vi "File_Application  Path INI Location.vi"() -> (0 "Path INI Location":path)   [LabVIEW 2015]
uses:
  <vilib>/Utility/sysdir.llb/System Directory Type.ctl
panel:
  in  "Name of System (Save as Default)":string="MySystem.ini"
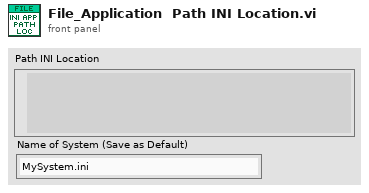
[diagram p1: front panel]
types:
  T1 = typedef "System Directory Type.ctl" = i32
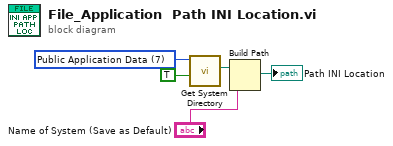
[diagram p0: block diagram]
diagram:
  w1 = T1 7 items=["User Home"=0, "User Desktop"=1, "User Documents"=2, "User Application Data"=3, "User Preferences"=4, "User Temporary"=5, "Public Documents"=6, "Public Application Data"=7, "Public Preferences"=8, "Public Cache"=13, "System Core Libraries"=9, "System Installed Libraries"=10, "Application Files"=11, "Boot Volume Root"=12] ("system directory type")
  n1 = call <vilib>:"Get System Directory.vi"("create directory if not found? (F)"=TRUE, "system directory type"=w1) -> ("system directory"=w3:path)  [unwired: 9 in]
  n2 = Build Path(base path=w3, name or relative path="Name of System (Save as Default)") -> (appended path=→"Path INI Location":path)
